vi "Append to Command.vi"(7 "Command Line Options":T1, 8 "error in (no error)":errorcluster, 10 "Parameter":string, 11 "MPLab in":refnum<class "MPLab.lvclass">) -> (0 "error out":errorcluster, 3 "MPLab out":refnum<class "MPLab.lvclass">)   [LabVIEW 2018, in "MPLab.lvlib" / "MPLab.lvclass"]
uses:
  MPLab.lvclass
  Custom Controls/Command Line Options.ctl
  MPLab.lvclass/MPLab.ctl
panel:
  in  "Command Line Strings":string[](array[string])=["-b", "-e", "-f", "-i", "-k", "-l", "-m", "-p", "-t", "-y"]
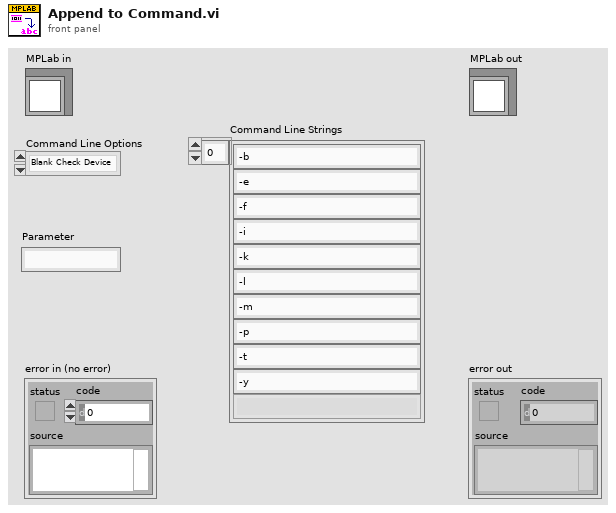
[diagram p1: front panel]
types:
  T1 = typedef "MPLab.lvlib/MPLab.lvclass/Command Line Options.ctl" = enum16{"Blank Check Device", "Erase Flash Device", "Hex File", "Display Device ID", "Display File Checksum", "Low Voltage Programming", "Memory Region", "Part", "Tool", "Verify Device"}
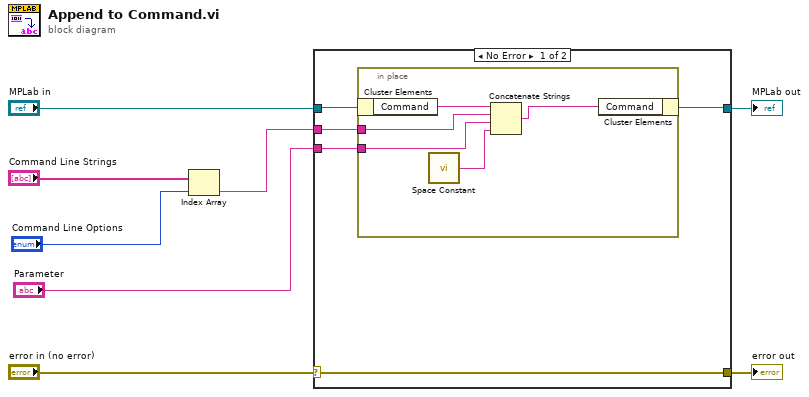
[diagram p0: block diagram]
diagram:
  n1 = Index Array(array="Command Line Strings", index="Command Line Options") -> (element=w2:string)
  n2 = case shown="No Error" "error in (no error)" {
    selector: "error in (no error)" -> [w13 w20]
    tunnel: [w13 w20] -> w7
    tunnel: [w11 w19] -> w5
    tunnel: "MPLab in" -> [w12 w19]
    tunnel: w2 -> [w10 _]
    tunnel: "Parameter" -> [w9 _]
    frame No Error {
      n3 = in-place {
        in-place-border: w10 -> [w16]
        in-place-border: w9 -> [w15]
        n4 = in-place-cluster #1(w12) -> ("Command"=w18:string)
        n5 = call <vilib>:"Space Constant.vi"() -> ("String"=w14:string)
        n6 = Concatenate Strings(w18, w16, w15, w14) -> (w17:string)
        n7 = in-place-cluster #1("Command"=w17) -> (w11:refnum<class "MPLab.lvclass">)
      }
    }
    frame Error {
    }
  }
  "error out" <- w7
  "MPLab out" <- w5
